vi "1motorPosCtrl (SubVI).vi"(6 "reset Encoder":bool, 7 "Motor ID":T1, 8 "Error In":errorcluster, 10 "Target (deg)":dbl, 11 "TitanQuad in":refnum<class "TitanQuad.lvclass">) -> (0 "error out":errorcluster, 1 "Cluster":cluster{"Target (deg)":dbl, "Enc (deg)":dbl}, 2 "Enc (deg)":dbl, 3 "TitanQuad out":refnum<class "TitanQuad.lvclass">)   [LabVIEW 2020]
uses:
  <vilib>/CISH Robotics/L4VMX TitanQuad/Motor ID.ctl
  <vilib>/CISH Robotics/L4VMX TitanQuad/TitanQuad.lvclass
  <vilib>/addons/control/pid/pid.llb/PID (DBL).vi
  <vilib>/addons/control/pid/NI_PID_pid.lvlib
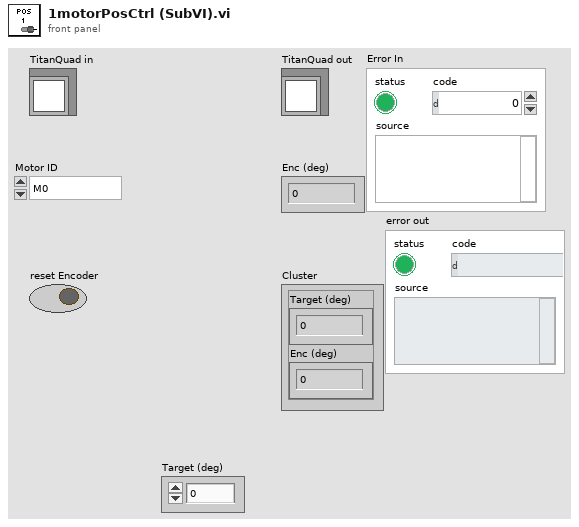
[diagram p1: front panel]
types:
  T1 = typedef "TitanQuad.lvlib/TitanQuad.lvclass/Motor ID.ctl" = enum16{"M0", "M1", "M2", "M3"}
  T2 = cluster{"proportional gain (Kc)":dbl, "integral time (Ti, min)":dbl, "derivative time (Td, min)":dbl}
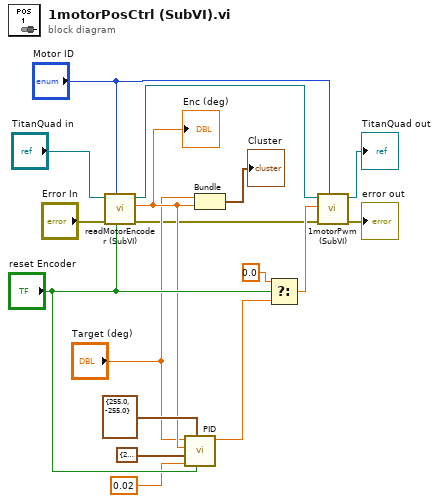
[diagram p0: block diagram]
diagram:
  n1 = call "readMotorEncoder (SubVI).vi"("reset Encoder"="reset Encoder", "Motor ID"="Motor ID", "Error In"="Error In", "TitanQuad in"="TitanQuad in") -> ("Error Out"=w2:errorcluster, "Enc (deg)"=w11:dbl, "TitanQuad out"=w5:refnum<class "TitanQuad.lvclass">)  [unwired: 5 in]
  "Enc (deg)" <- w11
  n2 = call-poly <vilib>:"PID.vi"("reinitialize? (F)"="reset Encoder", "output range"=cluster{"output high":dbl, "output low":dbl} {"output high"=255.0, "output low"=-255.0}, "dt (s)"=0.02, "PID gains"=T2 {"proportional gain (Kc)"=2.0, "integral time (Ti, min)"=0.0, "derivative time (Td, min)"=0.0005}, "process variable"=w11, "setpoint"="Target (deg)") -> ("output"=w15:dbl)  [unwired: 4 in, 1 out]
  n3 = Bundle("Target (deg)"="Target (deg)", "Enc (deg)"=w11) -> (→"Cluster":cluster{"Target (deg)":dbl, "Enc (deg)":dbl})  [unwired: 1 in]
  n4 = Select(t=0.0, s="reset Encoder", f=w15) -> (s? t:f=w17:dbl)
  n5 = call "1motorPwm (SubVI).vi"("Motor ID"="Motor ID", "error in (no error)"=w2, "motorPwmSpeed"=w17, "TitanQuad in"=w5) -> ("error out"=→"error out":errorcluster, "TitanQuad out"=→"TitanQuad out":refnum<class "TitanQuad.lvclass">)  [unwired: 6 in]
